vi "LOERN_MessageWithUI.vi"(0 "XRef":T6, 1 "Message In":T5, 2 "State In":T1={"Inputs"=1, "SelectedIndex"=0, "ClassInfo"=[], "Parallel VI"=refnum}) -> (14 "Message Out":T5, 15 "Reply":T4, 16 "Fatal Error Out":T3, 17 "State Out":T1={"Inputs"=1, "SelectedIndex"=0, "ClassInfo"=[], "Parallel VI"=refnum})   [LabVIEW 2016]
uses:
  <vilib>/XNodeSupport/XNodeXNodeRef.ctl
  <vilib>/XNodeSupport/XNodeString.ctl
  LOERN_State.ctl
  LOERN_ClassInfo.ctl
  <vilib>/XNodeSupport/XNodeStringArray.ctl
  <vilib>/XNodeSupport/XNodeErrorCluster.ctl
  <vilib>/XNodeSupport/NI_XNodeSupport.lvlib
  LV Object Event Registration Node.xnode
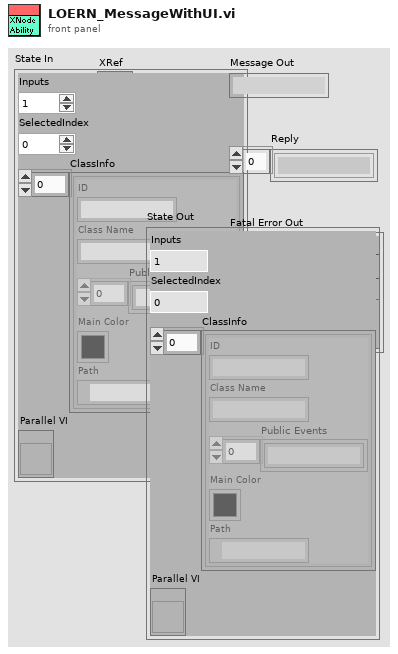
[diagram p1: front panel]
types:
  T1 = typedef "LV Object Event Registration Node.xnode/LOERN_State.ctl" = cluster{"Inputs":u16, "SelectedIndex":i16, "ClassInfo":T2[], "Parallel VI":refnum<vi>}
  T2 = typedef "LV Object Event Registration Node.xnode/LOERN_ClassInfo.ctl" = cluster{"ID":string, "Class Name":string, "Public Events":string[], "Main Color":u32, "Path":path}
  T3 = typedef "NI_XNodeSupport.lvlib/XNodeErrorCluster.ctl" = errorcluster
  T4 = typedef "NI_XNodeSupport.lvlib/XNodeStringArray.ctl" = T5[]
  T5 = typedef "NI_XNodeSupport.lvlib/XNodeString.ctl" = string
  T6 = typedef "NI_XNodeSupport.lvlib/XNodeXNodeRef.ctl" = refnum<vi>
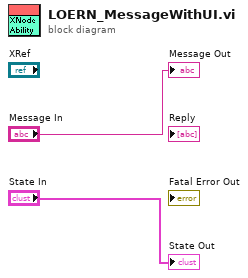
[diagram p0: block diagram]
diagram:
  "Message Out" <- "Message In"
  "State Out" <- "State In"
